vi "HoppingStep(Nonlinear-XZEnhancedSampleCurr2nd).vi"() -> ()   [LabVIEW 2014]
uses:
  <vilib>/Platform/TimedLoop/XDataNode/timing_clust.ctl
  <vilib>/Platform/TimedLoop/XDataNode/nitl_modes.ctl
  <vilib>/Platform/TimedLoop/XDataNode/wakeup.ctl
  <vilib>/rvi/Emulation/niFpgaGetClockAttributes.vi
  <vilib>/rvi/Emulation/niFpgaSctlEmulationGetInTimedLoop.vi
  <vilib>/rvi/Emulation/niFpgaEmulationReportErrorSimple.vi
  <vilib>/rvi/eio/common/nirviEmuTemplateMethod_errors.vi
  <vilib>/rvi/Emulation/niFpgaProcessEmulError.vi
  <vilib>/rvi/Emulation/niFpgaCriticalErrorInLSC.vi
  <vilib>/rvi/interface/RandomDataEmulation/niFpgaRandomDataHandleErrors.vi
  <vilib>/eio/EIONode/EIONode.xnode
  <vilib>/Platform/TimedLoop/XDataNode/XDataNode.xnode
  <vilib>/rvi/DataTransferAndStorage/Container/XNode/niFpgaContainer.xnode
  <vilib>/rvi/interface/RandomDataEmulation/nirviRandomDataFpgaReadWriteTemplate.vi
  <vilib>/Platform/TimedLoop/XDataNode/XDNodeRunTimeDep.lvlib
panel:
  in  "ZLimitFluctuationRange":i16
  in  "CheckNum":i16
  in  "BottomSleep us":i16=80
  in  "UpperSleep us":i16=150
  out "ZRealPos":i16
  in  "RelativeWithdraw":i16
  out "Waveform Chart":i32(graph)
  in  "stop":bool
  out "Z":i32(graph)
  in  "ZOffset":i16
  in  "XOffset":i16
  in  "XNum":i16
  in  "XStepIndex":i16
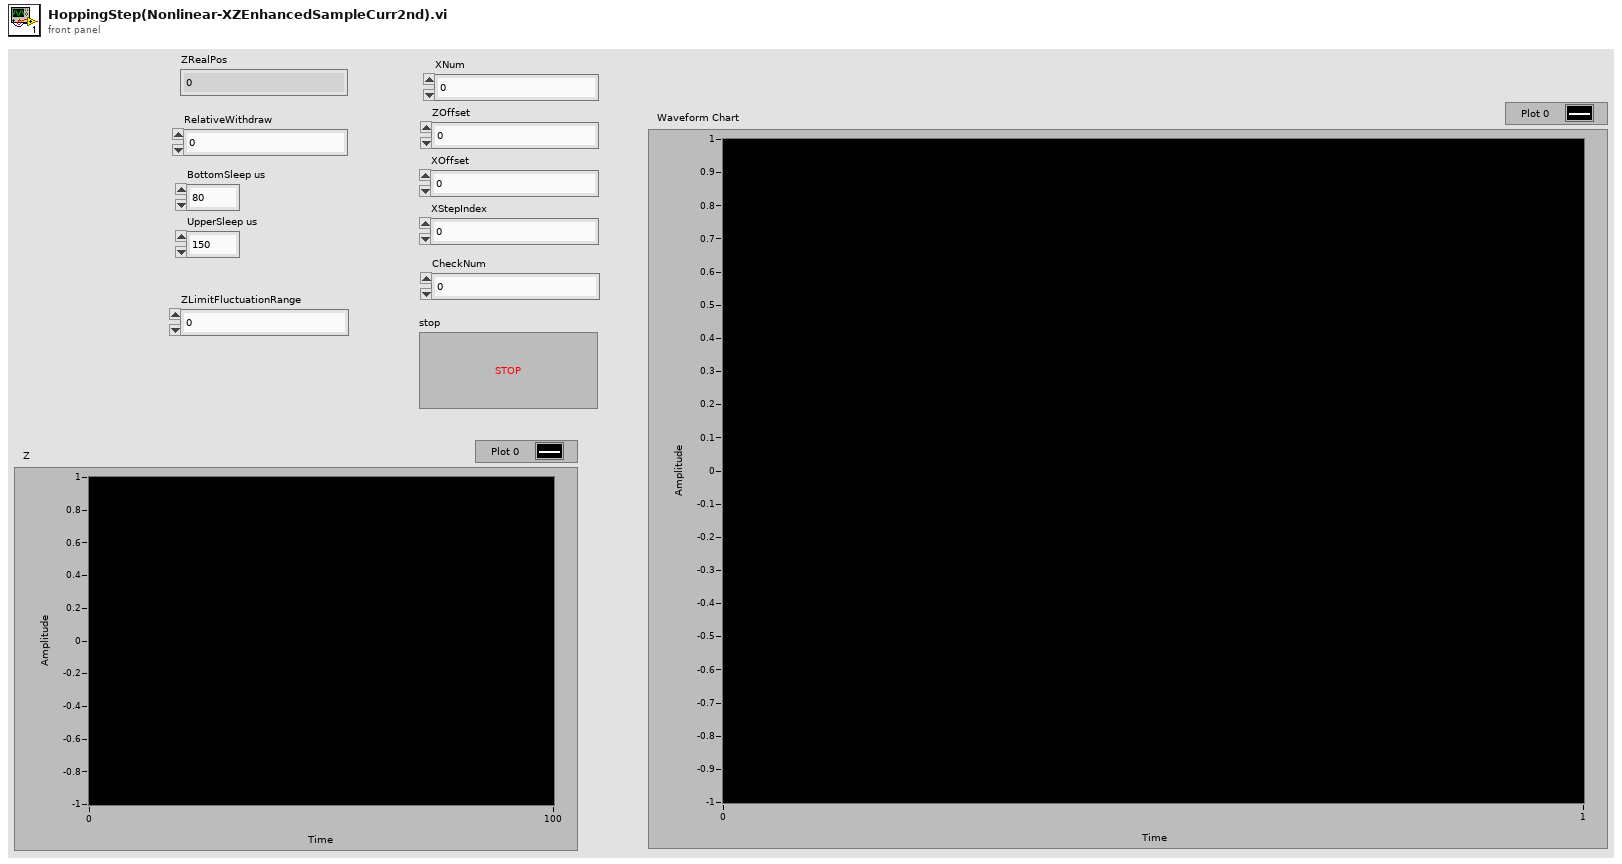
[diagram p1: front panel]
types:
  T1 = typedef "XDNodeRunTimeDep.lvlib/timing_clust.ctl" = cluster{"Expected End [f-1]":u64, "Actual End [f-1]":u64, "Finished Late? [f-1]":bool, "Expected End [i-1]":u64, "Actual End [i-1]":u64, "Finished Late? [i-1]":bool, "Expected Start [i]":u64, "Actual Start [i]":u64, "Expected Start [f]":u64, "Actual Start [f]":u64, "Source Name":string, "Structure Name":string, "Period":i64, "Deadline":i64, "Offset":i64, "Start":i64, "Priority":i32, "Timeout":i32, "Mode":T2, "Wakeup Reason":T3, "Error":errorcluster, "Source Type":string, "Secondary Source Type":string, "Global End Time":u64, "Global Start Time":u64, "Frame Duration":u64, "Iteration Duration":u64, "Assigned CPU":i32, "I/O Scan Engine Mode":u32}
  T2 = typedef "XDNodeRunTimeDep.lvlib/nitl_modes.ctl" = enum32{"No Change", "Process missed periods, maintain original phase", "Discard missed periods, maintain original phase", "Process missed periods, ignore original phase", "Discard missed periods, ignore original phase"}
  T3 = typedef "XDNodeRunTimeDep.lvlib/wakeup.ctl" = enum32{"Normal", "Aborted", "Asynchronous wakeup", "Timing source error", "Timed loop error", "Timeout"}
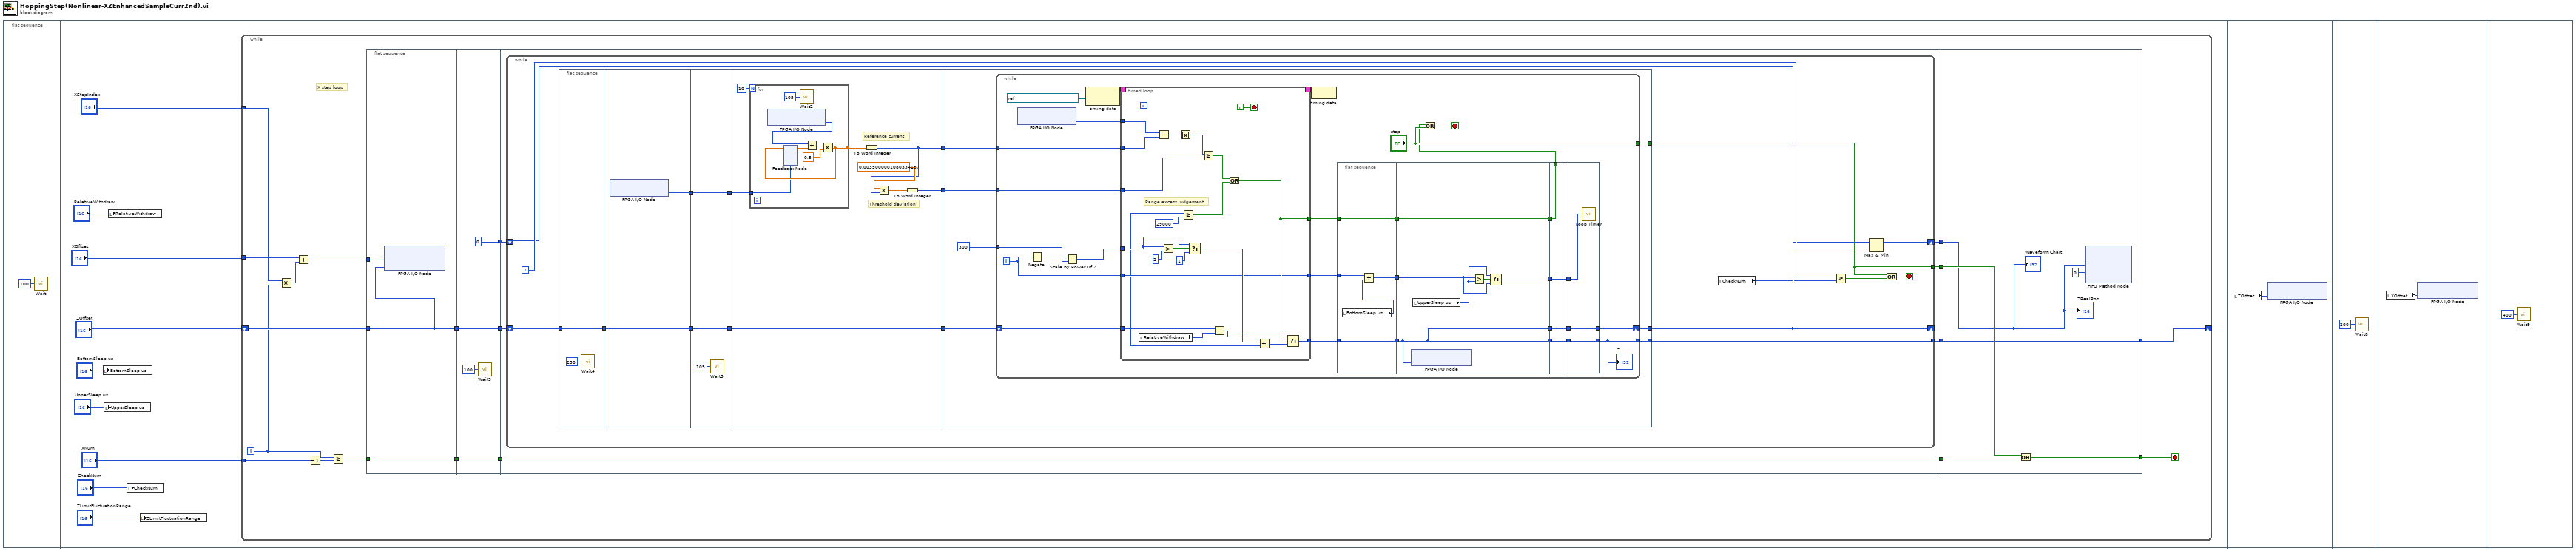
[diagram p0: block diagram]
diagram:
  n1 = flat-sequence {
    frame #0 {
      n2 = call "Wait"("Count(mSec)"=u32 100 ("Count(uSec)")) -> ()  [unwired: 1 out]
    }
    frame #1 {
      n3 = local write "BottomSleep us"("BottomSleep us") -> ()
      n4 = local write "UpperSleep us"("UpperSleep us") -> ()
      n5 = local write "RelativeWithdraw"("RelativeWithdraw") -> ()
      n6 = local write "CheckNum"("CheckNum") -> ()
      n7 = local write "ZLimitFluctuationRange"("ZLimitFluctuationRange") -> ()
      n8 = while {
        tunnel: "XNum" -> [w22]
        tunnel: "XStepIndex" -> [w23]
        shift-right: [w13] -> _
        shift-left: "ZOffset" -> [w24]
        tunnel: "XOffset" -> [w20]
        i -> [w12]
        stop <- w28 stop-if-true
        # "X step loop"
        n9 = Multiply(x=w23, y=w12) -> (x*y=w27:i32)
        n10 = Add(x=w20, y=w27) -> (x+y=w11:i32)
        n11 = Decrement(x=w22) -> (x-1=w21:i16)
        n12 = Greater Or Equal?(x=w12, y=w21) -> (x >= y?=w18:bool)
        n13 = flat-sequence {
          tunnel: [w33] -> w19
          tunnel: w24 -> [w33]
          tunnel: w18 -> [w32]
          tunnel: [w32] -> w16
          tunnel: w11 -> [w31]
          tunnel: [w37] -> w30
          tunnel: [i16 0] -> w26
          tunnel: w19 -> [w37]
          tunnel: [w34] -> w17
          tunnel: w16 -> [w34]
          tunnel: w30 -> [w43]
          tunnel: [w42] -> w29
          tunnel: w26 -> [w41]
          tunnel: [w40] -> w25
          tunnel: w17 -> [w39]
          tunnel: [w39] -> w15
          tunnel: [w38] -> w14
          tunnel: [w170] -> w28
          tunnel: w25 -> [w165]
          tunnel: w29 -> [w168]
          tunnel: w15 -> [w167]
          tunnel: w14 -> [w166]
          tunnel: [w166] -> w13
          frame #0 {
            n14 = xnode "FPGA I/O Node"("Connector0/AO2"=w31, "Connector0/AO0"=w33) -> ()  [unwired: 2 in, 2 out]
          }
          frame #1 {
            n15 = call "Wait3"("Count(uSec)"=u32 100) -> ()  [unwired: 1 out]
          }
          frame #2 {
            n16 = while {
              tunnel: [w47] -> w42
              shift-right: [w46] -> _
              shift-left: w43 -> [w58]
              shift-right: [w59] -> w40
              shift-left: w41 -> [w60]
              tunnel: [w50] -> w38
              i -> [w61]
              stop <- w49 stop-if-true
              n17 = flat-sequence {
                tunnel: w58 -> [w63]
                tunnel: [w63] -> w44
                tunnel: [w65] -> w53
                tunnel: [w64] -> w51
                tunnel: w44 -> [w65]
                tunnel: [w68] -> w54
                tunnel: w53 -> [w68]
                tunnel: [w66] -> w52
                tunnel: w51 -> [w66]
                tunnel: [w70] -> w57
                tunnel: [w69] -> w56
                tunnel: [w76] -> w55
                tunnel: w54 -> [w76]
                tunnel: w52 -> [w74]
                tunnel: [w88] -> w47
                tunnel: [w87] -> w46
                tunnel: w57 -> [w90]
                tunnel: w56 -> [w89]
                tunnel: w55 -> [w85]
                tunnel: [w84] -> w50
                frame #0 {
                  n18 = call "Wait4"("Count(uSec)"=u32 250) -> ()  [unwired: 1 out]
                }
                frame #1 {
                  n19 = xnode "FPGA I/O Node"() -> ("Connector0/AI1"=w64:i16)  [unwired: 1 in, 1 out]
                }
                frame #2 {
                  n20 = call "Wait5"("Count(uSec)"=u32 105) -> ()  [unwired: 1 out]
                }
                frame #3 {
                  # "Threshold deviation"
                  # "Reference current"
                  n21 = for {
                    N: 10 -> [_]
                    tunnel: [w78] -> w71
                    tunnel: w74 -> [w77]
                    n22 = xnode "FPGA I/O Node"() -> ("Connector0/AI1"=w79:i16)  [unwired: 1 in, 1 out]
                    n23 = feedback #1(w77) -> (w82:sgl)
                    n24 = call "Wait2"("Count(uSec)"=u32 105) -> ()  [unwired: 1 out]
                    n25 = Add(x=w79, y=w82) -> (x+y=w81:sgl)
                    n26 = Multiply(x=w81, y=sgl 0.5) -> (x*y=w78:sgl)
                    n27 = feedback-in #1(w78) -> ()
                  }
                  n28 = To Word Integer(number=w71) -> (16bit integer=w70:i16)
                  n29 = Multiply(x=sgl 0.0035, y=w70) -> (x*y=w72:sgl)
                  n30 = To Word Integer(number=w72) -> (16bit integer=w69:i16)
                }
                frame #4 {
                  n31 = while {
                    tunnel: w90 -> [w112]
                    tunnel: w89 -> [w114]
                    tunnel: ["stop"] -> w88
                    shift-right: [w106] -> w87
                    shift-left: w85 -> [w109]
                    tunnel: i16 300 -> [w96]
                    tunnel: [w91] -> w84
                    i -> [w94]
                    stop <- w116 stop-if-true
                    n32 = xnode "FPGA I/O Node"() -> ("Connector0/AI1"=w113:i16)  [unwired: 1 in, 1 out]
                    n33 = Negate(x=w94) -> (-x=w97:i32)
                    n34 = Scale By Power Of 2(n=w97, x=w96) -> (x*2^n=w95:i16)
                    n35 = node-c288(refnum<k21> "40 MHz Onboard Clock" ("Source Name")) -> (w119:T1)
                    n36 = timed-loop {
                      timing: w119 -> [_]
                      timing-out: [_] -> w118
                      tunnel: w112 -> [w156]
                      tunnel: w114 -> [w141]
                      tunnel: w113 -> [w157]
                      tunnel: [w152] -> w110
                      tunnel: [w151] -> w108
                      tunnel: w109 -> [w140]
                      tunnel: w95 -> [w144]
                      tunnel: [w146] -> w98
                      tunnel: w94 -> [w146]
                      stop <- TRUE stop-if-true
                      # "Range excess judgement"
                      n37 = local read "RelativeWithdraw"() -> (w138:i16)
                      n38 = Subtract(x=w157, y=w156) -> (x-y=w142:i16)
                      n39 = Greater?(x=w144, y=i16 2) -> (0:w143:bool)
                      n40 = Absolute Value(x=w142) -> (abs(x)=w155:i16)
                      n41 = Greater Or Equal?(x=w140, y=i16 29000) -> (x >= y?=w153:bool)
                      n42 = Select(t=w144, s=w143, f=1) -> (s? t:f=w147:i32)
                      n43 = Greater Or Equal?(x=w155, y=w141) -> (x >= y?=w154:bool)
                      n44 = Subtract(x=w140, y=w138) -> (x-y=w139:i32)
                      n45 = Or(x=w154, y=w153) -> (x .or. y?=w151:bool)
                      n46 = Add(x=w147, y=w140) -> (x+y=w149:i32)
                      n47 = Select(t=w139, s=w151, f=w149) -> (s? t:f=w152:i32)
                    }
                    n48 = node-c288(w118) -> ()
                    n49 = flat-sequence {
                      tunnel: [w124] -> w111
                      tunnel: w110 -> [w124]
                      tunnel: w108 -> [w123]
                      tunnel: [w123] -> w107
                      tunnel: [w121] -> w99
                      tunnel: w98 -> [w122]
                      tunnel: w111 -> [w125]
                      tunnel: [w125] -> w105
                      tunnel: w107 -> [w130]
                      tunnel: [w130] -> w103
                      tunnel: [w128] -> w100
                      tunnel: w99 -> [w127]
                      tunnel: [w125] -> w92
                      tunnel: w105 -> [w134]
                      tunnel: [w134] -> w104
                      tunnel: w103 -> [w133]
                      tunnel: [w133] -> w102
                      tunnel: [w132] -> w101
                      tunnel: w100 -> [w132]
                      tunnel: [w131] -> w93
                      tunnel: w92 -> [w131]
                      tunnel: w104 -> [w137]
                      tunnel: [w137] -> w106
                      tunnel: w101 -> [w136]
                      tunnel: [w135] -> w91
                      tunnel: w93 -> [w135]
                      frame #0 {
                        n50 = local read "BottomSleep us"() -> (w120:i16)
                        n51 = Add(x=w122, y=w120) -> (x+y=w121:i32)
                      }
                      frame #1 {
                        n52 = xnode "FPGA I/O Node"("Connector0/AO0"=w125) -> ()  [unwired: 1 in, 1 out]
                        n53 = local read "UpperSleep us"() -> (w126:i16)
                        n54 = Greater?(x=w127, y=w126) -> (0:w129:bool)
                        n55 = Select(t=w126, s=w129, f=w127) -> (s? t:f=w128:i32)
                      }
                      frame #2 {
                      }
                      frame #3 {
                        n56 = call "Loop Timer"("Count(uSec)"=w136) -> ()  [unwired: 1 out]
                      }
                    }
                    n57 = Or(x=w102, y="stop") -> (x .or. y?=w116:bool)
                    "Z" <- w91
                  }
                }
              }
              n58 = local read "CheckNum"() -> (w45:i16)
              n59 = Greater Or Equal?(x=w61, y=w45) -> (x >= y?=w48:bool)
              n60 = Max & Min(x=w60, y=w46) -> (max(x,y)=w59:i32)  [unwired: 1 out]
              n61 = Compound Arithmetic op=OR(w47, w48) -> (w49:bool)
            }
          }
          frame #3 {
            n62 = Or(x=w168, y=w167) -> (x .or. y?=w170:bool)
            n63 = xnode ("FIFO Method Node")("Element"=w165, "Timeout"=0) -> ()  [unwired: 1 in, 2 out]
            "Waveform Chart" <- w165
            "ZRealPos" <- w165
          }
        }
      }
    }
    frame #2 {
      n64 = local read "ZOffset"() -> (w171:i16)
      n65 = xnode "FPGA I/O Node"("Connector0/AO0"=w171) -> ()  [unwired: 1 in, 1 out]
    }
    frame #3 {
      n66 = call "Wait8"("Count(uSec)"=u32 200) -> ()  [unwired: 1 out]
    }
    frame #4 {
      n67 = local read "XOffset"() -> (w173:i16)
      n68 = xnode "FPGA I/O Node"("Connector0/AO2"=w173) -> ()  [unwired: 1 in, 1 out]
    }
    frame #5 {
      n69 = call "Wait9"("Count(uSec)"=u32 400) -> ()  [unwired: 1 out]
    }
  }
